vi "鼠标离开颜色写入.vi"(4 "error in (no error)":errorcluster, 5 "Value":cluster{"Color Box":u32, "Color Box 2":u32}[](array[cluster]) caption="鼠标离开颜色写入", 6 "Container State":T2, 7 "Display State In":T1) -> (0 "error out":errorcluster, 3 "Display State Out":T1)   [LabVIEW 2011, in "ChangeColorBtn.xctl"]
uses:
  ChangeColorBtn.xctl
  <vilib>/_xctls/Container State.ctl
  State 1.ctl
  <vilib>/_xctls/XControlSupport.lvlib
panel:
  # "Replace the Value Control below with a Control of desired type.\nDo not remove this Control or the others from the connector pane.\nDo not change the connector pane pattern.\nThe Value control should always be the third terminal from top on the input side in the connector pane."
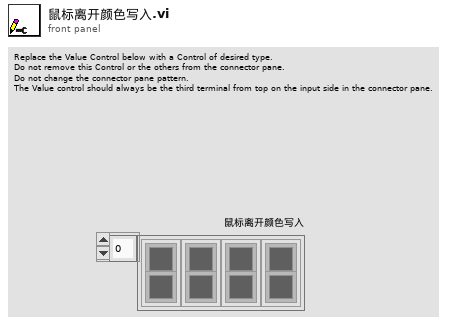
[diagram p1: front panel]
types:
  T1 = typedef "ChangeColorBtn.xctl/State 1.ctl" = cluster{"鼠标进入标题":string, "鼠标离开标题":string, "鼠标进入颜色":cluster{"Color Box":u32, "Color Box 2":u32}[], "鼠标离开颜色":cluster{"Color Box":u32, "Color Box 2":u32}[]}
  T2 = typedef "XControlSupport.lvlib/Container State.ctl" = cluster{"Indicator?":bool, "Run Mode?":bool, " Refnum":refnum<vi>}
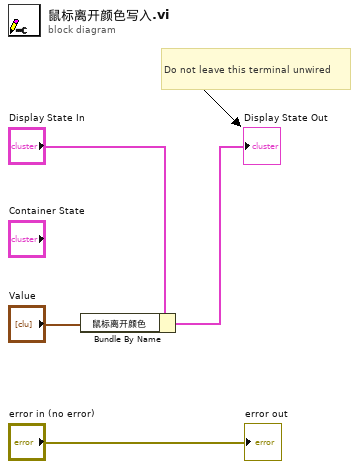
[diagram p0: block diagram]
diagram:
  # "Do not leave this terminal unwired"
  n1 = Bundle By Name(cluster="Display State In", "鼠标离开颜色"="Value") -> (→"Display State Out":T1)
  "error out" <- "error in (no error)"
